vi "sub_bits_to_symbols.vi"(8 "symbol map":cdb[](array[numeric]), 11 "bits":i16[](array[numeric])) -> (3 "symbols":cdb[](array[numeric]))   [LabVIEW 2014]
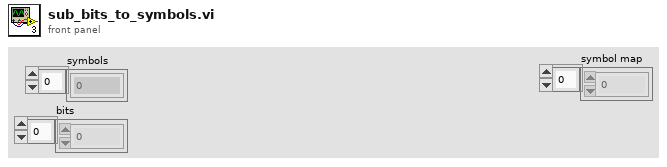
[diagram p1: front panel]
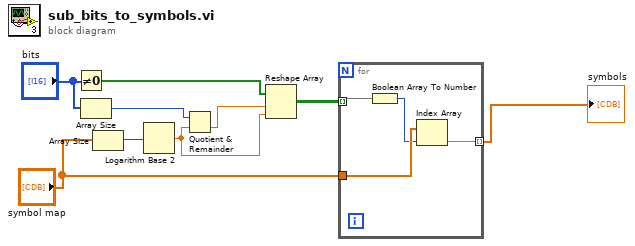
[diagram p0: block diagram]
diagram:
  n1 = Not Equal To 0?(x="bits") -> (x != 0?=w6:bool[])
  n2 = Array Size(array="bits") -> (size(s)=w7:i32)
  n3 = Array Size(array="symbol map") -> (size(s)=w9:i32)
  n4 = Logarithm Base 2(1:w9) -> (0:w4:dbl)
  n5 = Quotient & Remainder(x=w7, y=w4) -> (floor(x/y)=w5:dbl)  [unwired: 1 out]
  n6 = Reshape Array(w6, w5, w4) -> (w3:bool[][])
  n7 = for {
    tunnel: w3 -> [w13] mode=indexing
    tunnel: "symbol map" -> [w12]
    tunnel: [w10] -> w1 mode=indexing
    n8 = Boolean Array To Number(Boolean array=w13) -> (number=w11:u32)
    n9 = Index Array(array=w12, index=w11) -> (element=w10:cdb)
  }
  "symbols" <- w1
